vi "Main.vi"(11 "Module Admin":refnum<class "Delacor_lib_QMH_Module Admin.lvclass">) -> ()   [LabVIEW 2020, in "Pruebas.lvlib"]
doc: "This template is based off of the Queued Message Handler design pattern and the Queued Message Handler project template that ships with LabVIEW.\n\nThe main difference is that the queue is private to this module and communication between modules is performed via Broadcast and Request events.\n\nRequest events are wrapped in public API methods and are handled in the Event Handling Loop (EHL) of this VI. Any module can register for Broadcast events sent by this module. The EHL generates messages based on user interface actions.\n\nThe Message Handling Loop (MHL) processes messages generated by the EHL, or by other messages. The messages are string values, so new messages can be added easily to the Message Cases case structure in the MHL. Each message cluster can also provide an optional value for Message Data, which is a variant that can be converted to whatever message-specific data is required.\n_____\nBased on Delacor QMH Project Template 5.0.0.82."
uses:
  Pruebas.lvlib
  <vilib>/Delacor/Delacor QMH/Libraries/Module Admin_class/Delacor_lib_QMH_Module Admin.lvclass
  Module Data--cluster.ctl
  <vilib>/Delacor/Delacor QMH/Libraries/Message Queue_class/Delacor_lib_QMH_Message Queue.lvclass/Delacor_lib_QMH_Message Queue.ctl
  Stop Argument--cluster.ctl
  <vilib>/Delacor/Delacor QMH/Libraries/Module Admin_class/Delacor_lib_QMH_Module Admin.lvclass/Delacor_lib_QMH_Module Admin.ctl
  Mostrar en Subpanel Argument--cluster.ctl
  <vilib>/Utility/miscctls.llb/LVPointTypeDef.ctl
  <vilib>/Delacor/Delacor QMH/Libraries/Message Queue_class/Delacor_lib_QMH_Enqueue Message (Single).vi
  <vilib>/Delacor/Delacor QMH/Libraries/Module Admin_class/Delacor_lib_QMH_Get External Launch.vi
  <vilib>/Utility/error.llb/Error Cluster From Error Code.vi
  <vilib>/ErrorRing/Error Ring.xnode
  <vilib>/Delacor/Delacor QMH/Libraries/Message Queue_class/Delacor_lib_QMH_Message Queue.lvclass
panel:
  out "Señales Debug Ref":refnum<vi>[](array[refnum])
  out "Señales de Prueba Ref":refnum<vi>[](array[refnum])
  in  "Modulación Corrientes":dbl min=0.0 max=50.0 step=5.0 format="%#_g %%"
  in  "Modulación T002":dbl min=0.0 max=90.0 step=5.0 format="%#_g %%"
  in  "Modulación T001":dbl min=0.0 max=90.0 step=5.0 format="%#_g %%"
  in  "DebugMode":bool
  in  "Fases 3 y 4":bool
  in  "Fases 1 y 2":bool
  in  "Cojinetes":bool
  in  "Corriente de Armadura":dbl min=0.0 max=2000.0 step=50.0 format="%#_g A"
  in  "Corriente de Campo":dbl min=0.0 max=3.0 step=0.1 format="%#_g A"
  in  "Tensión Batería":dbl min=0.0 max=340.0 step=10.0 format="%#_g V"
  in  "Tensión Generador":dbl min=0.0 max=340.0 step=10.0 format="%#_g V"
  in  "Habilitar Señales de Prueba":bool
  out "error out":errorcluster
  out "Status":string
  # "Panel de Pruebas"
  # "Depuración [Modulación PWMs]"
  # "Simular Sobretemperatura"
  # "Amperímetros y Voltímetros"
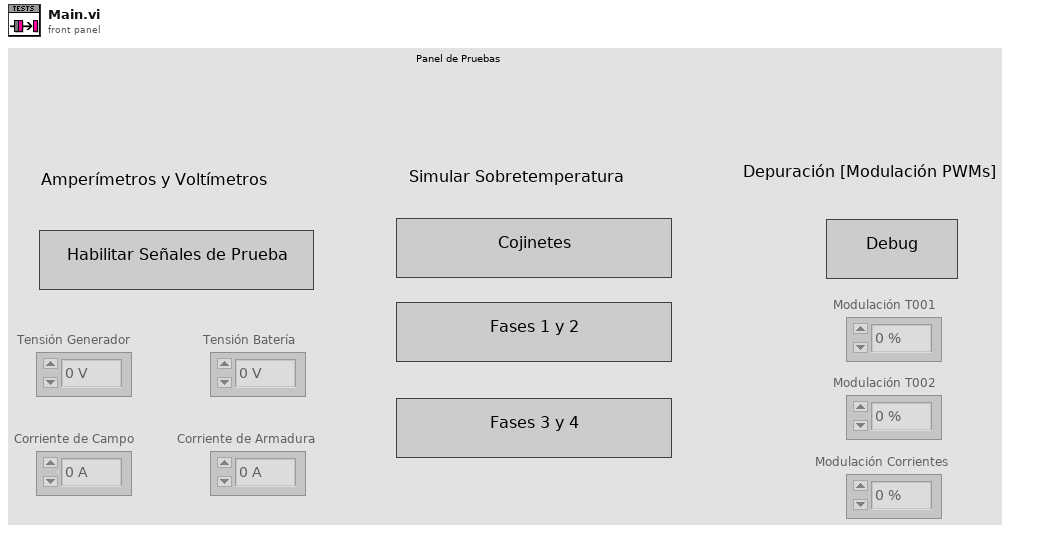
[diagram p1: front panel]
types:
  T1 = typedef "Pruebas.lvlib/Request Events--cluster.ctl" = cluster{"Stop Module":refnum<user-event>, "Show Panel":refnum<user-event>, "Hide Panel":refnum<user-event>, "Get Module Execution Status":refnum<user-event>, "Show Diagram":refnum<user-event>, "Mostrar en Subpanel":refnum<user-event>}
  T2 = typedef "Pruebas.lvlib/Module Data--cluster.ctl" = cluster{"Status":string}
  T3 = enum32{"invalid lock state", "Not Locked", "Locked (No Password)", "Password-protected"}
  T4 = typedef "Pruebas.lvlib/Stop Argument--cluster.ctl" = cluster{"Origin":string, "Exit via Stop Module Req?":bool, "Wait for Module to stop?":bool}
  T5 = typedef "Pruebas.lvlib/Mostrar en Subpanel Argument--cluster.ctl" = cluster{"Subpanel Ref":refnum<vi>}
  T6 = typedef "LVPointTypeDef.ctl" = cluster{"Horizontal":i16, "Vertical":i16}
  T7 = enum32{"Invalid", "Standard", "Closed", "Hidden", "Minimized", "Maximized"}
  T8 = enum8{"Enabled", "Disabled", "Disabled and Grayed Out"}
  T9 = cluster{"Cojinetes":bool, "Fases 1 y 2":bool, "Fases 3 y 4":bool}
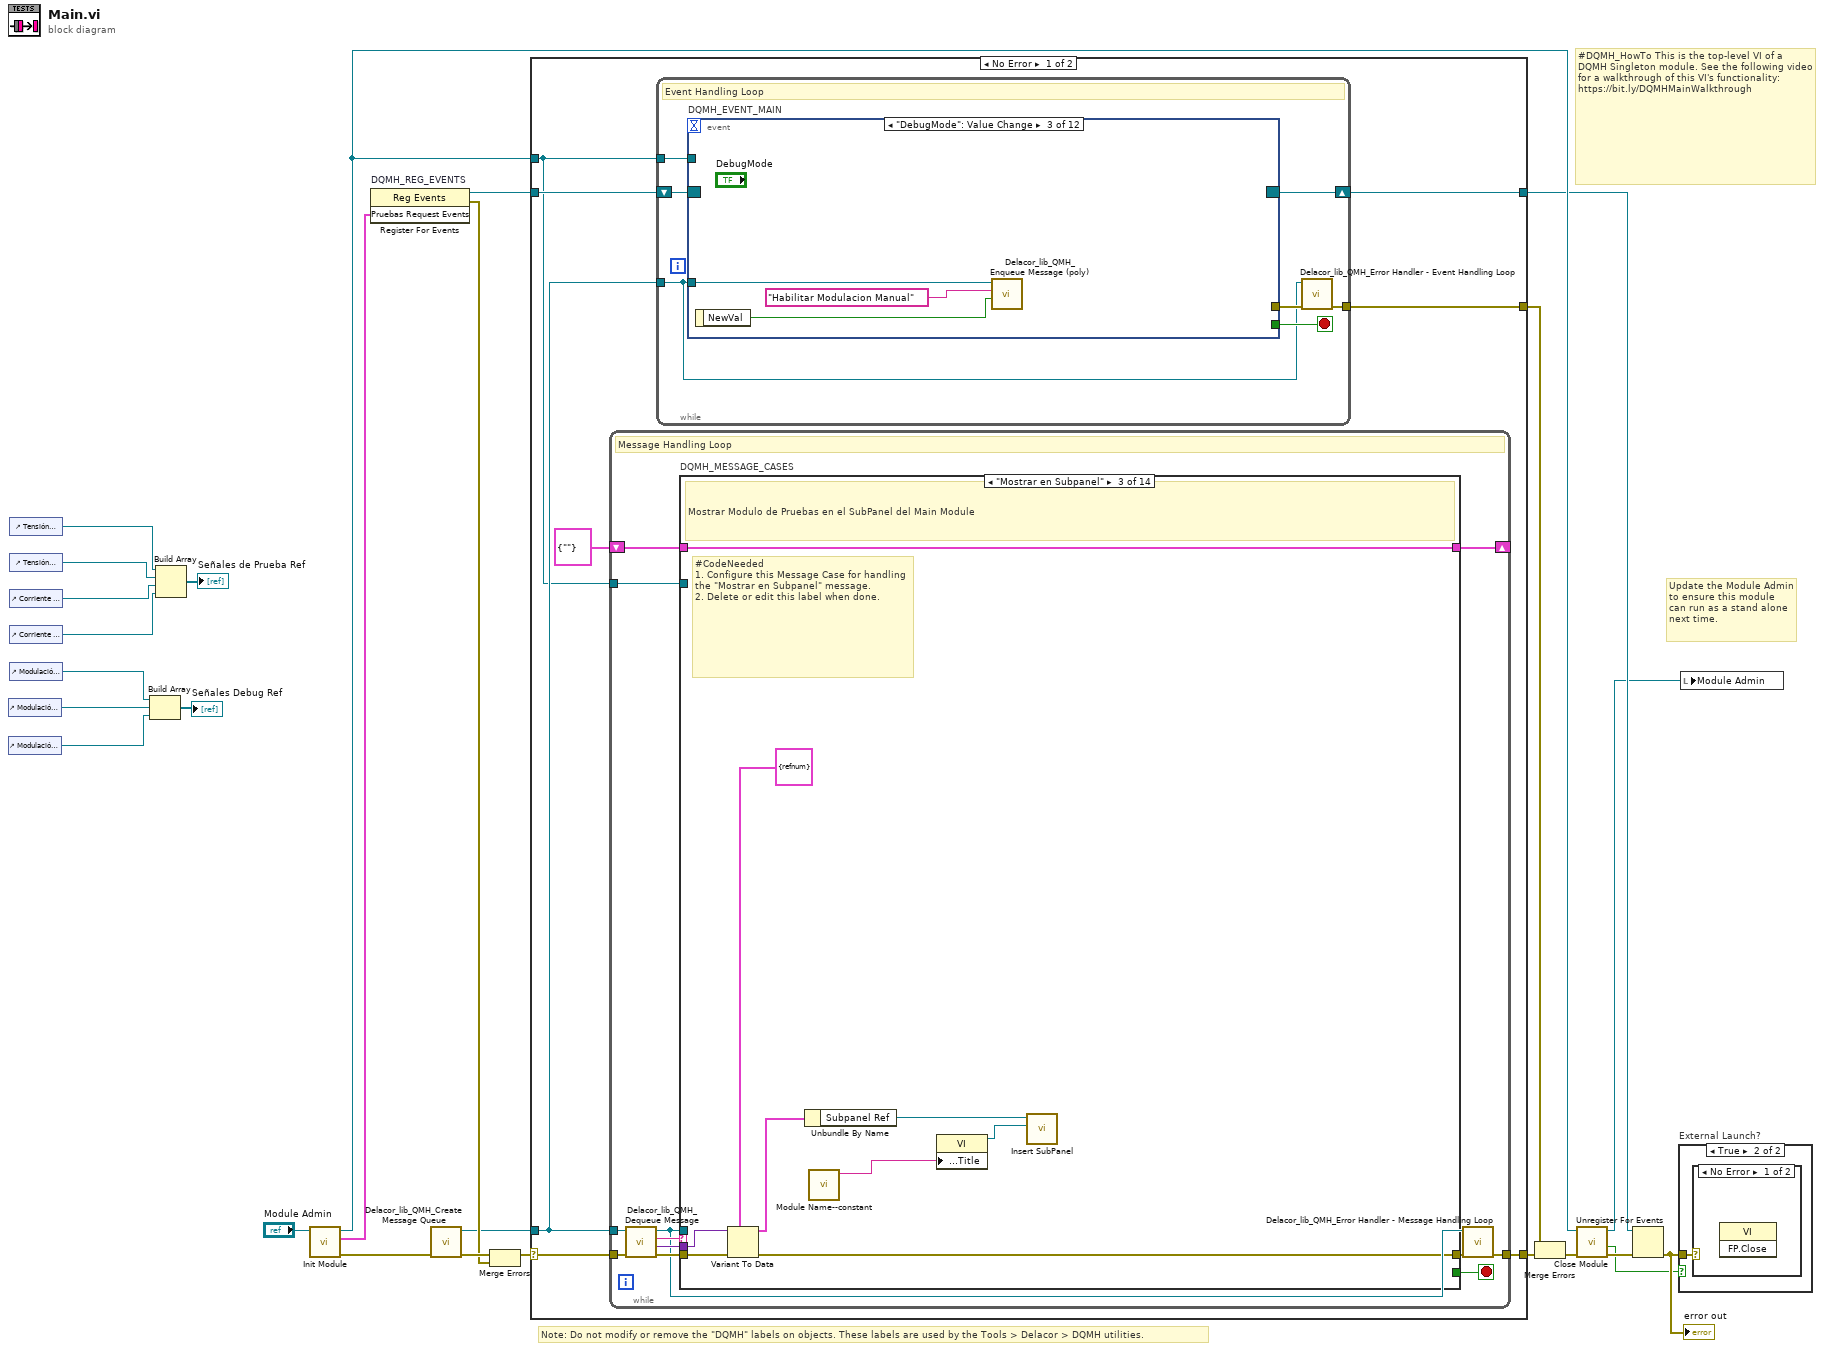
[diagram p0: block diagram]
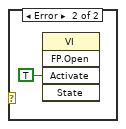
[diagram p3: hidden frame]
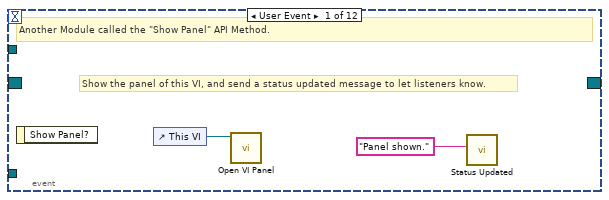
[diagram p4: hidden frame]
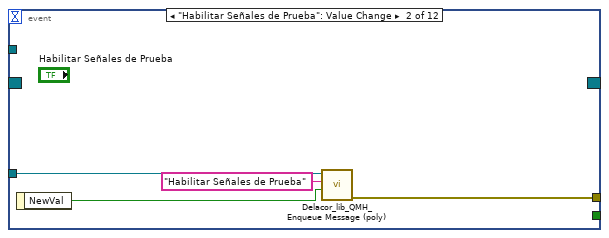
[diagram p5: hidden frame]
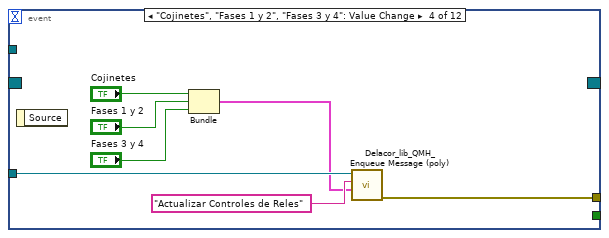
[diagram p6: hidden frame]
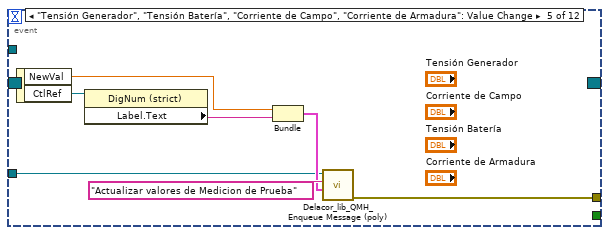
[diagram p7: hidden frame]
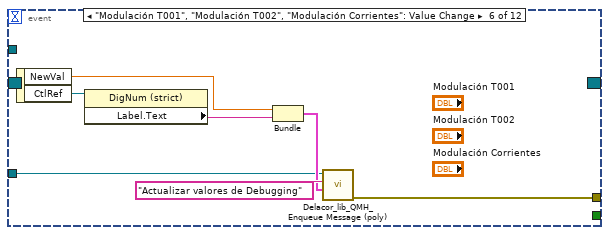
[diagram p8: hidden frame]
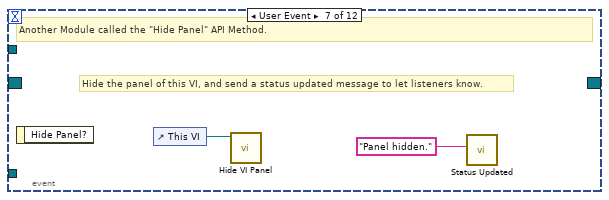
[diagram p9: hidden frame]
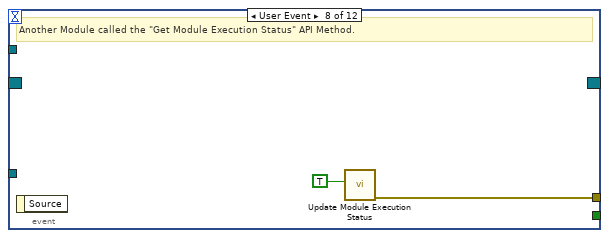
[diagram p10: hidden frame]
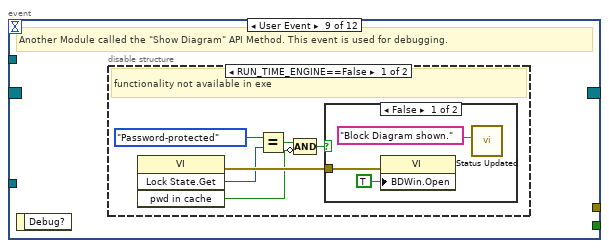
[diagram p11: hidden frame]
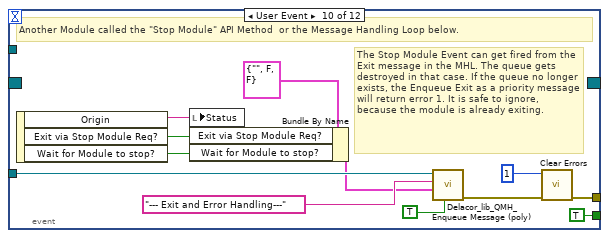
[diagram p14: hidden frame]
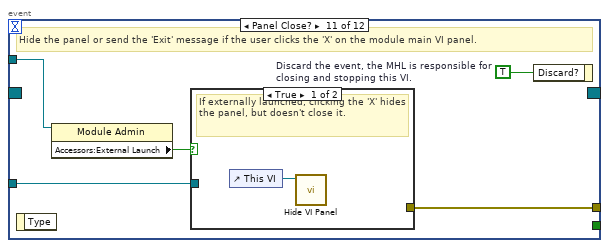
[diagram p15: hidden frame]
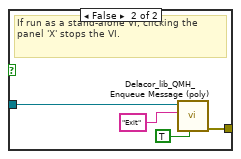
[diagram p16: hidden frame]
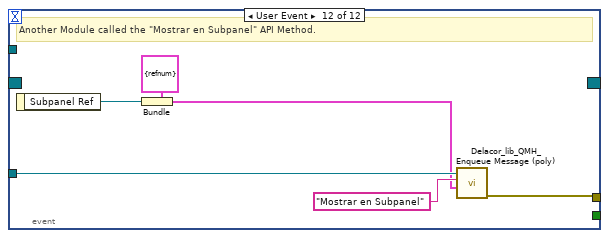
[diagram p17: hidden frame]
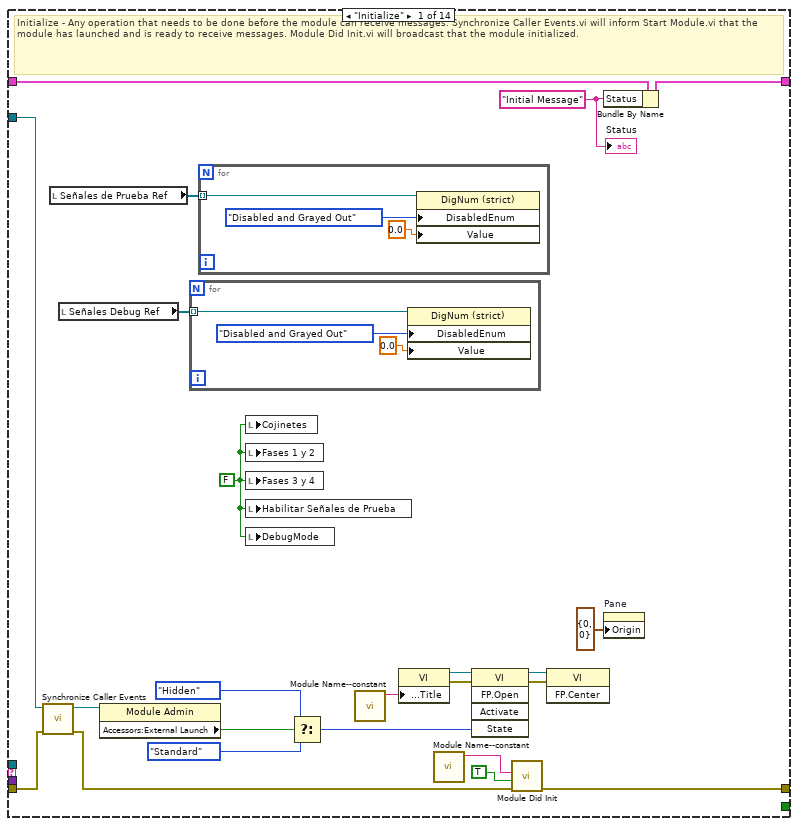
[diagram p18: hidden frame]
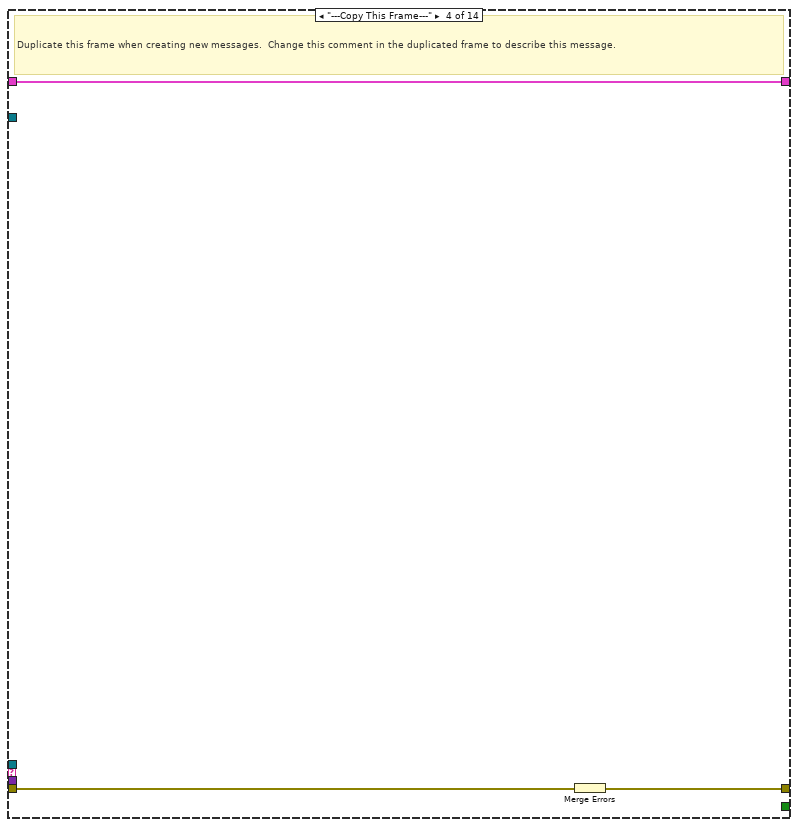
[diagram p20: hidden frame]
diagram:
  # "#DQMH_HowTo This is the top-level VI of a DQMH Singleton module. See the following video for a walkthrough of this VI's functionality: https://bit.ly/DQMHMainWalkthrough"
  # "Note: Do not modify or remove the \"DQMH\" labels on objects. These labels are used by the Tools > Delacor > DQMH utilities."
  # "Update the Module Admin to ensure this module can run as a stand alone next time."
  n1 = control-ref of="Modulación Corrientes"() -> (w3:refnum<vi>)
  n2 = control-ref of="Modulación T002"() -> (w2:refnum<vi>)
  n3 = control-ref of="Tensión Generador"() -> (w9:refnum<vi>)
  n4 = control-ref of="Tensión Batería"() -> (w8:refnum<vi>)
  n5 = control-ref of="Corriente de Campo"() -> (w7:refnum<vi>)
  n6 = control-ref of="Corriente de Armadura"() -> (w6:refnum<vi>)
  n7 = control-ref of="Modulación T001"() -> (w4:refnum<vi>)
  n8 = Build Array(w4, w3, w2) -> (→"Señales Debug Ref":refnum<vi>[])
  n9 = Build Array(w9, w8, w7, w6) -> (→"Señales de Prueba Ref":refnum<vi>[])
  n10 = call "Init Module.vi"("Singleton Module Admin in"="Module Admin") -> ("error out"=w25:errorcluster, "Pruebas Request Events"=w14:T1, "Singleton Module Admin out"=w17:refnum<class "Delacor_lib_QMH_Module Admin.lvclass">)  [unwired: 8 in]
  n11 = register-events "DQMH_REG_EVENTS"(w14) -> (reference out=w15:refnum<event-registration>, error out=w18:errorcluster)  [unwired: 2 in]
  n12 = call <vilib>:"Delacor_lib_QMH_Create Message Queue.vi"("error in"=w25) -> ("error out"=w20:errorcluster, "Message Queue"=w13:refnum<class "Delacor_lib_QMH_Message Queue.lvclass">)  [unwired: 9 in]
  n13 = Merge Errors(w20, w18) -> (w19:errorcluster)
  n14 = case shown="No Error" w19 {
    selector: w19 -> [w32 w309]
    tunnel: [w34 w308] -> w26
    tunnel: [w31 w314] -> w16
    tunnel: w15 -> [w29 w314]
    tunnel: w13 -> [w28 w307]
    tunnel: [w33 _] -> w23
    tunnel: w17 -> [w27 w310]
    frame No Error {
      n15 = while {
        tunnel: w28 -> [w115]
        shift-right: [w119] -> _
        shift-left: T2 {"Status"=""} ("Data Cluster") -> [w120]
        tunnel: w32 -> [w123]
        tunnel: [w121] -> w34
        tunnel: w27 -> [w113]
        stop <- w118 stop-if-true
        # "Message Handling Loop"
        n16 = call-dynamic "Delacor_lib_QMH_Dequeue Message.vi"("error in"=w123, "Message Queue in"=w115) -> ("error out"=w122:errorcluster, "Message Data"=w116:variant, "Message"=w117:string, "Message Queue out"=w114:refnum<class "Delacor_lib_QMH_Message Queue.lvclass">)  [unwired: 6 in]
        n17 = case "DQMH_MESSAGE_CASES" shown="\"Mostrar en Subpanel\"" w117 {
          selector: w117 -> [_ _ _ _ _ _ _ _ _ _ _ _ _ w294]
          tunnel: w114 -> [_ _ _ _ _ _ _ _ _ w247 _ w264 w286 _]
          tunnel: w122 -> [w145 w155 w164 w167 w172 w189 w201 w216 w232 _ w253 w271 w292 w296]
          tunnel: [w143 w155 w162 w166 w175 w192 w204 w219 w235 w246 w252 w267 w289 w297] -> w124
          tunnel: w120 -> [w134 w154 w163 w165 w174 w191 w203 w218 w234 w248 w250 w266 w285 w295]
          tunnel: [w133 w154 w163 w165 w174 w191 w203 w218 w234 w248 w250 w266 w285 w295] -> w119
          tunnel: [_ _ _ _ _ _ _ _ _ _ _ _ w284 _] -> w118
          tunnel: w116 -> [_ _ w161 _ w173 w190 w202 w217 w233 _ _ w265 w283 _]
          tunnel: w113 -> [w135 _ _ _ _ _ _ _ _ _ _ w263 w278 _]
          frame "Initialize" {
            w125 = FALSE ("DebugMode")
            w128 = "Initial Message" ("Initial Message")
            # "Initialize - Any operation that needs to be done before the module can receive messages. Synchronize Caller Events.vi will inform Start Module.vi that the module has launched and is ready to receive messages. Module Did Init.vi will broadcast that the module initialized."
            n18 = call "Synchronize Caller Events.vi"("error in (no error)"=w145, "Singleton Module Admin in"=w135) -> ("error out"=w144:errorcluster, "Singleton Module Admin out"=w130:refnum<class "Delacor_lib_QMH_Module Admin.lvclass">)  [unwired: 8 in]
            n19 = local read "Señales de Prueba Ref"() -> (w127:refnum<vi>[])
            n20 = local read "Señales Debug Ref"() -> (w126:refnum<vi>[])
            n21 = property class="Module Admin"(reference=w130) -> ("Accessors:External Launch"=w139:bool)  [unwired: 1 in, 2 out]
            n22 = for {
              tunnel: w126 -> [w150] mode=indexing
              n23 = property class="DigNum (strict)"(reference=w150, "DisabledEnum"=T8."Disabled and Grayed Out" ("Disabled"), "Value"=0.0) -> ()  [unwired: 1 in, 2 out]
            }
            n24 = for {
              tunnel: w127 -> [w153] mode=indexing
              n25 = property class="DigNum (strict)"(reference=w153, "DisabledEnum"=T8."Disabled and Grayed Out" ("Disabled"), "Value"=0.0) -> ()  [unwired: 1 in, 2 out]
            }
            n26 = local write "Cojinetes"(w125) -> ()
            n27 = local write "Fases 1 y 2"(w125) -> ()
            n28 = local write "Fases 3 y 4"(w125) -> ()
            n29 = local write "Habilitar Señales de Prueba"(w125) -> ()
            n30 = local write "DebugMode"(w125) -> ()
            n31 = Select(t=T7."Hidden" ("State"), s=w139, f=T7."Standard" ("State")) -> (s? t:f=w136:T7)
            n32 = call "Module Name--constant.vi"() -> ("Module Name"=w142:string)  [unwired: 11 in]
            n33 = property class="VI"("Front Panel.Title"=w142) -> (reference out=w141:refnum<vi>, error out=w147:errorcluster)  [unwired: 2 in]
            n34 = call "Module Name--constant.vi"() -> ("Module Name"=w131:string)  [unwired: 11 in]
            n35 = invoke class="VI" method="FP.Open"(reference=w141, error in=w147, "State"=w136) -> (reference out=w140:refnum<vi>, error out=w146:errorcluster)  [unwired: 2 in, 3 out]
            n36 = call "Module Did Init.vi"("error in (no error)"=w144, "Initialized?"=TRUE, "Origin"=w131) -> ("error out"=w143:errorcluster)  [unwired: 8 in]
            n37 = invoke class="VI" method="FP.Center"(reference=w140, error in=w146) -> ()  [unwired: 1 in, 3 out]
            n38 = Bundle By Name(cluster=w134, "Status"=w128) -> (w133:T2)
            n39 = property on="Pane" class="Pane"("Origin"=T6 {"Horizontal"=0, "Vertical"=0}) -> ()  [unwired: 2 in, 2 out]
            "Status" <- w128
          }
          frame "--- Module Specific ---" {
            # "Separator -- The following cases handle messages specific to this Module."
          }
          frame "Mostrar en Subpanel" {
            # "#CodeNeeded\n1. Configure this Message Case for handling the \"Mostrar en Subpanel\" message.\n2. Delete or edit this label when done."
            # "Mostrar Modulo de Pruebas en el SubPanel del Main Module"
            n40 = Variant To Data(error in=w164, type=T5 {"Subpanel Ref"=refnum} ("Mostrar en Subpanel Argument"), Variant=w161) -> (data=w159:T5, error out=w162:errorcluster)
            n41 = Unbundle By Name(w159) -> ("Subpanel Ref"=w158:refnum<vi>)
            n42 = call "Module Name--constant.vi"() -> ("Module Name"=w157:string)  [unwired: 11 in]
            n43 = property class="VI"("Front Panel.Title"=w157) -> (reference out=w156:refnum<vi>)  [unwired: 2 in, 1 out]
            n44 = call "Insert SubPanel.vi"("VI Ref"=w156, "Subpanel Ref"=w158) -> ()  [unwired: 9 in, 1 out]
          }
          frame "---Copy This Frame---" {
            # "Duplicate this frame when creating new messages.  Change this comment in the duplicated frame to describe this message."
            n45 = Merge Errors(w167) -> (w166:errorcluster)
          }
          frame "Habilitar Señales de Prueba" {
            # "Duplicate this frame when creating new messages.  Change this comment in the duplicated frame to describe this message."
            n46 = local read "Señales de Prueba Ref"() -> (w169:refnum<vi>[])
            n47 = Variant To Data(error in=w172, type=FALSE ("Habilitar Señales de Prueba 2"), Variant=w173) -> (data=w168:bool, error out=w171:errorcluster)
            n48 = case shown="True" w168 {
              tunnel: w169 -> [w177 w180]
              frame False {
                w176 = 0.0 ("Tensión Generador")
                n49 = for {
                  tunnel: w177 -> [w179] mode=indexing
                  n50 = property class="DigNum (strict)"(reference=w179, "DisabledEnum"=T8."Disabled and Grayed Out" ("Disabled")) -> ()  [unwired: 1 in, 2 out]
                }
                n51 = local write "Tensión Generador"(w176) -> ()
                n52 = local write "Tensión Batería"(w176) -> ()
                n53 = local write "Corriente de Campo"(w176) -> ()
                n54 = local write "Corriente de Armadura"(w176) -> ()
              }
              frame True {
                n55 = for {
                  tunnel: w180 -> [w182] mode=indexing
                  n56 = property class="DigNum (strict)"(reference=w182, "DisabledEnum"=T8."Enabled" ("Disabled")) -> ()  [unwired: 1 in, 2 out]
                }
              }
            }
            n57 = Merge Errors(w171) -> (w175:errorcluster)
          }
          frame "Actualizar valores de Medicion de Prueba" {
            # "Duplicate this frame when creating new messages.  Change this comment in the duplicated frame to describe this message."
            n58 = Variant To Data(error in=w189, type=cluster{"NewVal":dbl, "Label.Text":string} {"NewVal"=0.0, "Label.Text"=""} ("output cluster"), Variant=w190) -> (data=w187:cluster{"NewVal":dbl, "Label.Text":string}, error out=w184:errorcluster)
            n59 = Unbundle(w187) -> ("NewVal"=w186:dbl, "Label.Text"=w185:string)
            n60 = call "Valor de Medicion de Prueba Enviado.vi"("error in (no error)"=w184, "Nombre del Valor"=w185, "Valor"=w186) -> ("error out"=w183:errorcluster)  [unwired: 8 in]
            n61 = Merge Errors(w183) -> (w192:errorcluster)
          }
          frame "Actualizar valores de Debugging" {
            # "Duplicate this frame when creating new messages.  Change this comment in the duplicated frame to describe this message."
            n62 = Variant To Data(error in=w201, type=cluster{"NewVal":dbl, "Label.Text":string} {"NewVal"=0.0, "Label.Text"=""} ("output cluster"), Variant=w202) -> (data=w199:cluster{"NewVal":dbl, "Label.Text":string}, error out=w197:errorcluster)
            n63 = Unbundle(w199) -> ("NewVal"=w195:dbl, "Label.Text"=w196:string)
            n64 = Divide(x=w195, y=100.0) -> (x/y=w194:dbl)
            n65 = case shown="\"Modulación T001\"" w196 {
              tunnel: w194 -> [w206 w208 w210]
              frame "Modulación T002", Default {
                n66 = shared-variable-write(refnum<k21> "ni.var.psp://EmuGenV2/VariablesEmuGenV2/Mod T002 Debug" ("shared variable refnum in"), w206) -> ()  [unwired: 1 in, 2 out]
              }
              frame "Modulación Corrientes" {
                n67 = shared-variable-write(refnum<k21> "ni.var.psp://EmuGenV2/VariablesEmuGenV2/Mod Corriente Debug" ("shared variable refnum in"), w208) -> ()  [unwired: 1 in, 2 out]
              }
              frame "Modulación T001" {
                n68 = shared-variable-write(refnum<k21> "ni.var.psp://EmuGenV2/VariablesEmuGenV2/Mod T001 Debug" ("shared variable refnum in"), w210) -> ()  [unwired: 1 in, 2 out]
              }
            }
            n69 = call "Valor de Modulacion Debugging Enviado.vi"("error in (no error)"=w197, "Nombre"=w196, "Valor"=w195) -> ("error out"=w198:errorcluster)  [unwired: 8 in]
            n70 = Merge Errors(w198) -> (w204:errorcluster)
          }
          frame "Habilitar Modulacion Manual" {
            # "Duplicate this frame when creating new messages.  Change this comment in the duplicated frame to describe this message."
            n71 = local read "Señales Debug Ref"() -> (w213:refnum<vi>[])
            n72 = Variant To Data(error in=w216, type=FALSE ("Habilitar Señales de Prueba 2"), Variant=w217) -> (data=w212:bool, error out=w215:errorcluster)
            n73 = case shown="True" w212 {
              tunnel: w213 -> [w220 w223]
              frame False {
                n74 = for {
                  tunnel: w220 -> [w222] mode=indexing
                  n75 = property class="DigNum (strict)"(reference=w222, "DisabledEnum"=T8."Disabled and Grayed Out" ("Disabled")) -> ()  [unwired: 1 in, 2 out]
                }
              }
              frame True {
                n76 = for {
                  tunnel: w223 -> [w225] mode=indexing
                  n77 = property class="DigNum (strict)"(reference=w225, "DisabledEnum"=T8."Enabled" ("Disabled")) -> ()  [unwired: 1 in, 2 out]
                }
              }
            }
            n78 = shared-variable-write(refnum<k21> "ni.var.psp://EmuGenV2/VariablesEmuGenV2/Habilitar Debug" ("shared variable refnum in"), w212) -> ()  [unwired: 1 in, 2 out]
            n79 = Merge Errors(w215) -> (w219:errorcluster)
          }
          frame "Actualizar Controles de Reles" {
            # "Duplicate this frame when creating new messages.  Change this comment in the duplicated frame to describe this message."
            n80 = Variant To Data(error in=w232, type=T9 {"Cojinetes"=FALSE, "Fases 1 y 2"=FALSE, "Fases 3 y 4"=FALSE} ("output cluster"), Variant=w233) -> (data=w229:T9, error out=w231:errorcluster)
            n81 = Unbundle By Name(w229) -> ("Fases 3 y 4"=w228:bool, "Cojinetes"=w227:bool, "Fases 1 y 2"=w226:bool)
            n82 = call "Controles de relés de prueba actualizados.vi"("Fases 3 y 4"=w228, "Fases 1 y 2"=w226, "Cojinete"=w227) -> ()  [unwired: 8 in, 1 out]
            n83 = Merge Errors(w231) -> (w235:errorcluster)
          }
          frame "--- Exit and Error Handling---" {
            # "Separator - The following cases handle errors and exit messages."
            n84 = call-poly <vilib>:"Delacor_lib_QMH_Enqueue Message (poly).vi"("Message Data"=T4 {"Origin"="", "Exit via Stop Module Req?"=FALSE, "Wait for Module to stop?"=FALSE} ("Stop Argument"), "Message"="Exit", "Message Queue in"=w247) -> ("error out"=w246:errorcluster)  [unwired: 7 in, 1 out]
            n85 = shared-variable-write(refnum<k21> "ni.var.psp://EmuGenV2/VariablesEmuGenV2/Habilitar Debug" ("shared variable refnum in"), FALSE ("Habilitar Debug")) -> ()  [unwired: 1 in, 2 out]
            n86 = shared-variable-write(refnum<k21> "ni.var.psp://EmuGenV2/VariablesEmuGenV2/Mod T001 Debug" ("shared variable refnum in"), 0.0 ("Mod T001 Debug")) -> ()  [unwired: 1 in, 2 out]
            n87 = shared-variable-write(refnum<k21> "ni.var.psp://EmuGenV2/VariablesEmuGenV2/Mod T002 Debug" ("shared variable refnum in"), 0.0 ("Mod T002 Debug")) -> ()  [unwired: 1 in, 2 out]
            n88 = shared-variable-write(refnum<k21> "ni.var.psp://EmuGenV2/VariablesEmuGenV2/Mod Corriente Debug" ("shared variable refnum in"), 0.0 ("Mod Corriente Debug")) -> ()  [unwired: 1 in, 2 out]
          }
          frame "Simulate MHL Error" {
            # "#DQMH_HowTo The 'Simulate MHL Error' button  illustrates how the MHL handles errors. This event is instructional in nature and can be removed."
            # "Simulate an error occurring at the MHL"
            n89 = call "Module Name--constant.vi"() -> ("Module Name"=w249:string)  [unwired: 11 in]
            n90 = xnode "Error Ring"("parameter 0"=w249) -> ("error out"=w251:errorcluster)
            n91 = Merge Errors(w253, w251) -> (w252:errorcluster)
          }
          frame "Error" {
            # "#CodeRecommended - If you ever change the name of this \"Error\" message, you'll need to update the name in the Check Loop Error.vi as well."
            # "#CodeRecommended - If the module is running in standalone mode (External Launch = FALSE), this code will pop up an error dialog and call the 'Exit' message if an error occurs. Add more fine-grained error handling here."
            # "Error - Check the error message data and respond accordingly. This message is sent by the \"Error Handler\" VIs at the end of each loop in this application."
            n92 = property class="Module Admin"(reference=w263) -> ("Accessors:External Launch"=w262:bool)  [unwired: 1 in, 2 out]
            n93 = Variant To Data(error in=w271, type=errorcluster {"status"=FALSE, "code"=0, "source"=""} ("error constant"), Variant=w265) -> (data=w272:errorcluster, error out=w269:errorcluster)
            n94 = call "Module Name--constant.vi"() -> ("Module Name"=w261:string)  [unwired: 11 in]
            n95 = call "Error Reported.vi"("Additional Information"=w261, "Error"=w272) -> ()  [unwired: 9 in, 1 out]
            n96 = case shown="False" w262 {
              tunnel: [w277 _] -> w268
              tunnel: w264 -> [w275 _]
              tunnel: w272 -> [w276 _]
              frame False {
                # "If the module is running standalone, then pop up an error dialog and call the \"Exit\" message."
                n97 = call <vilib>:"Simple Error Handler.vi"("error in (no error)"=w276) -> ()  [unwired: 4 in, 5 out]
                n98 = call-poly <vilib>:"Delacor_lib_QMH_Enqueue Message (poly).vi"("Priority Message? (F)"=TRUE, "Message"="Exit", "Message Queue in"=w275) -> ("error out"=w277:errorcluster)  [unwired: 7 in, 1 out]
              }
              frame True {
                # "If the module was launched externally, calling the Error Reported broadcast VI is the only action performed by the \"Error\" message. The module's caller can then process the error appropriately."
              }
            }
            n99 = Merge Errors(w269, w268) -> (w267:errorcluster)
            n100 = local write "error out"(w267) -> ()
          }
          frame "Exit" {
            w282 = 91  # 91: not all Exit messages will have an argument
            w284 = TRUE  # Stop the VI
            # "Release the message queue reference"
            # "#CodeNeeded - Add any required cleanup code here"
            # "Exit - Exit the application."
            n101 = Variant To Data(error in=w292, type=T4 {"Origin"="", "Exit via Stop Module Req?"=FALSE, "Wait for Module to stop?"=FALSE} ("Stop Argument"), Variant=w283) -> (data=w280:T4, error out=w288:errorcluster)
            n102 = call <vilib>:"Clear Errors.vi"("error in (no error)"=w288, "specific error code to clear (0: all)"=w282) -> ("error out"=w291:errorcluster)  [unwired: 4 in, 1 out]
            n103 = control-ref of="This VI"() -> (w279:refnum<vi>)
            n104 = call-dynamic "Delacor_lib_QMH_Release Message Queue.vi"("error in"=w291, "Message Queue"=w286) -> ("error out"=w290:errorcluster)  [unwired: 9 in]
            n105 = call "Handle Exit.vi"("Stop Argument"=w280, "Admin in"=w278, "VI reference"=w279) -> ("error out"=w287:errorcluster)  [unwired: 7 in, 1 out]
            n106 = Merge Errors(w290, w287) -> (w289:errorcluster)
          }
          frame Default {
            # "'Default' case only runs if there is a message that isn't defined in any of the other cases.  Output a programming error."
            n107 = call "Module Name--constant.vi"() -> ("Module Name"=w293:string)  [unwired: 11 in]
            n108 = xnode "Error Ring"("parameter 0"=w294, "parameter 1"=w293) -> ("error out"=w298:errorcluster)
            n109 = Merge Errors(w296, w298) -> (w297:errorcluster)
          }
        }
        n110 = call-dynamic "Delacor_lib_QMH_Error Handler - Message Handling Loop.vi"("error in"=w124, "Message Queue in"=w114) -> ("dup error in"=w121:errorcluster)  [unwired: 8 in, 1 out]
      }
      n111 = while {
        tunnel: w28 -> [w35]
        shift-right: [w38] -> w31
        shift-left: w29 -> [w39]
        tunnel: [w40] -> w33
        tunnel: w27 -> [w36]
        stop <- w37 stop-if-true
        # "Event Handling Loop"
        n112 = event "DQMH_EVENT_MAIN" shown="[2] \"DebugMode\": Value Change" {
          selector: w39 -> [_ _ _ _ _ _ _ _ _ _ _ _]
          dyn-events: [_ _ _ _ _ _ _ _ _ _ _ _] -> w38
          timeout: _ -> [_ _ _ _ _ _ _ _ _ _ _ _]
          tunnel: [_ _ _ _ _ _ _ _ _ TRUE ("Discard?") _ _] -> w37
          tunnel: w35 -> [_ w47 w49 w57 w59 w66 _ _ _ w92 w99 w112]
          tunnel: [_ w46 _ w51 w58 w65 _ w75 _ w95 w101 w107] -> w41
          tunnel: w36 -> [_ _ _ _ _ _ _ _ _ _ w98 _]
          event User Event {
            # "Show the panel of this VI, and send a status updated message to let listeners know."
            # "Another Module called the \"Show Panel\" API Method."
            n113 = event-data() -> ()  [unwired: 1 in, 1 out]
            n114 = control-ref of="This VI"() -> (w43:refnum<vi>)
            n115 = call "Open VI Panel.vi"("VI"=w43) -> ()  [unwired: 10 in, 1 out]
            n116 = call "Status Updated.vi"("Status"="Panel shown." ("format string")) -> ()  [unwired: 10 in, 1 out]
          }
          event "Habilitar Señales de Prueba": Value Change {
            n117 = event-data() -> ("NewVal"=w44:bool)  [unwired: 1 in]
            n118 = call-poly <vilib>:"Delacor_lib_QMH_Enqueue Message (poly).vi"("Message Data"=w44, "Message"="Habilitar Señales de Prueba", "Message Queue in"=w47) -> ("error out"=w46:errorcluster)  [unwired: 7 in, 1 out]
          }
          event "DebugMode": Value Change {
            n119 = event-data() -> ("NewVal"=w48:bool)  [unwired: 1 in]
            n120 = call-poly <vilib>:"Delacor_lib_QMH_Enqueue Message (poly).vi"("Message Data"=w48, "Message"="Habilitar Modulacion Manual", "Message Queue in"=w49) -> ()  [unwired: 7 in, 2 out]
          }
          event "Cojinetes", "Fases 1 y 2", "Fases 3 y 4": Value Change {
            n121 = event-data() -> ()  [unwired: 1 in, 1 out]
            n122 = Bundle("Cojinetes"="Cojinetes", "Fases 1 y 2"="Fases 1 y 2", "Fases 3 y 4"="Fases 3 y 4") -> (w52:T9)  [unwired: 1 in]
            n123 = call-poly <vilib>:"Delacor_lib_QMH_Enqueue Message (poly).vi"("Message Data"=w52, "Message"="Actualizar Controles de Reles", "Message Queue in"=w57) -> ("error out"=w51:errorcluster)  [unwired: 7 in, 1 out]
          }
          event "Tensión Generador", "Tensión Batería", "Corriente de Campo", "Corriente de Armadura": Value Change {
            n124 = event-data() -> ("NewVal"=w62:dbl, "CtlRef"=w64:refnum<vi>)  [unwired: 1 in]
            n125 = property class="DigNum (strict)"(reference=w64) -> ("Label.Text"=w61:string)  [unwired: 1 in, 2 out]
            n126 = Bundle("NewVal"=w62, "Label.Text"=w61) -> (w60:cluster{"NewVal":dbl, "Label.Text":string})  [unwired: 1 in]
            n127 = call-poly <vilib>:"Delacor_lib_QMH_Enqueue Message (poly).vi"("Message Data"=w60, "Message"="Actualizar valores de Medicion de Prueba", "Message Queue in"=w59) -> ("error out"=w58:errorcluster)  [unwired: 7 in, 1 out]
          }
          event "Modulación T001", "Modulación T002", "Modulación Corrientes": Value Change {
            n128 = event-data() -> ("NewVal"=w69:dbl, "CtlRef"=w71:refnum<vi>)  [unwired: 1 in]
            n129 = property class="DigNum (strict)"(reference=w71) -> ("Label.Text"=w68:string)  [unwired: 1 in, 2 out]
            n130 = Bundle("NewVal"=w69, "Label.Text"=w68) -> (w67:cluster{"NewVal":dbl, "Label.Text":string})  [unwired: 1 in]
            n131 = call-poly <vilib>:"Delacor_lib_QMH_Enqueue Message (poly).vi"("Message Data"=w67, "Message"="Actualizar valores de Debugging", "Message Queue in"=w66) -> ("error out"=w65:errorcluster)  [unwired: 7 in, 1 out]
          }
          event User Event {
            # "Hide the panel of this VI, and send a status updated message to let listeners know."
            # "Another Module called the \"Hide Panel\" API Method."
            n132 = event-data() -> ()  [unwired: 1 in, 1 out]
            n133 = control-ref of="This VI"() -> (w73:refnum<vi>)
            n134 = call "Hide VI Panel.vi"("VI"=w73) -> ()  [unwired: 10 in, 1 out]
            n135 = call "Status Updated.vi"("Status"="Panel hidden." ("format string")) -> ()  [unwired: 10 in, 1 out]
          }
          event User Event {
            # "Another Module called the \"Get Module Execution Status\" API Method."
            n136 = event-data() -> ()  [unwired: 1 in, 1 out]
            n137 = call "Update Module Execution Status.vi"("Running?"=TRUE) -> ("error out"=w75:errorcluster)  [unwired: 10 in]
          }
          event User Event {
            # "Another Module called the \"Show Diagram\" API Method. This event is used for debugging."
            n138 = event-data() -> ()  [unwired: 1 in, 1 out]
            n139 = disable-structure shown="RUN_TIME_ENGINE==False" {
              frame condition #0 (active) {
                # "functionality not available in exe"
                n140 = invoke class="VI" method="Lock State.Get"() -> (error out=w81:errorcluster, "Get Lock State"=w80:T3, "pwd in cache"=w77:bool)  [unwired: 4 in, 1 out]
                n141 = Equal?(x=T3."Password-protected", y=w80) -> (x = y?=w78:bool)
                n142 = Compound Arithmetic op=AND(w78, invert w77) -> (w76:bool)
                n143 = case shown="False" w76 {
                  tunnel: w81 -> [w84 _]
                  frame False {
                    n144 = property class="VI"(error in=w84, "BDWin.Open"=TRUE ("Block Diagram Window:Open")) -> ()  [unwired: 1 in, 2 out]
                    n145 = call "Status Updated.vi"("Status"="Block Diagram shown." ("format string")) -> ()  [unwired: 10 in, 1 out]
                  }
                  frame True {
                    # "Password-protected VI, and the password is not in the cache. Do not show the diagram."
                  }
                }
              }
              frame condition #1 {
              }
            }
          }
          event User Event {
            # "The Stop Module Event can get fired from the Exit message in the MHL. The queue gets destroyed in that case. If the queue no longer exists, the Enqueue Exit as a priority message will return error 1. It is safe to ignore, because the module is already exiting."
            # "Another Module called the \"Stop Module\" API Method  or the Message Handling Loop below."
            n146 = event-data() -> ("Origin"=w91:string, "Exit via Stop Module Req?"=w87:bool, "Wait for Module to stop?"=w86:bool)  [unwired: 1 in]
            n147 = local write "Status"(w91) -> ()
            n148 = Bundle By Name(cluster=T4 {"Origin"="", "Exit via Stop Module Req?"=FALSE, "Wait for Module to stop?"=FALSE} ("Stop Argument"), "Exit via Stop Module Req?"=w87, "Wait for Module to stop?"=w86) -> (w85:T4)
            n149 = call-poly <vilib>:"Delacor_lib_QMH_Enqueue Message (poly).vi"("Priority Message? (F)"=TRUE, "Message Data"=w85, "Message"="--- Exit and Error Handling---", "Message Queue in"=w92) -> ("error out"=w96:errorcluster)  [unwired: 6 in, 1 out]
            n150 = call <vilib>:"Clear Errors.vi"("error in (no error)"=w96, "specific error code to clear (0: all)"=1) -> ("error out"=w95:errorcluster)  [unwired: 4 in, 1 out]
          }
          event Panel Close? {
            w100 = TRUE  # Discard the event, the MHL is responsible for closing and stopping this VI.
            # "Hide the panel or send the 'Exit' message if the user clicks the 'X' on the module main VI panel."
            n151 = event-data() -> ()  [unwired: 1 in, 1 out]
            n152 = property class="Module Admin"(reference=w98) -> ("Accessors:External Launch"=w97:bool)  [unwired: 1 in, 2 out]
            n153 = case shown="True" w97 {
              tunnel: w99 -> [_ w105]
              tunnel: [_ w106] -> w101
              frame True {
                # "If externally launched, clicking the 'X' hides the panel, but doesn't close it."
                n154 = control-ref of="This VI"() -> (w102:refnum<vi>)
                n155 = call "Hide VI Panel.vi"("VI"=w102) -> ()  [unwired: 10 in, 1 out]
              }
              frame False {
                # "If run as a stand-alone VI, clicking the panel 'X' stops the VI."
                n156 = call-poly <vilib>:"Delacor_lib_QMH_Enqueue Message (poly).vi"("Priority Message? (F)"=TRUE, "Message"="Exit", "Message Queue in"=w105) -> ("error out"=w106:errorcluster)  [unwired: 7 in, 1 out]
              }
            }
            n157 = event-data("Discard?"=w100) -> ()  [unwired: 1 in, 1 out]
          }
          event User Event {
            # "Another Module called the \"Mostrar en Subpanel\" API Method."
            n158 = event-data() -> ("Subpanel Ref"=w108:refnum<vi>)  [unwired: 1 in]
            n159 = Bundle(cluster=T5 {"Subpanel Ref"=refnum} ("Mostrar en Subpanel Argument"), "Subpanel Ref"=w108) -> (w109:T5)
            n160 = call-poly <vilib>:"Delacor_lib_QMH_Enqueue Message (poly).vi"("Message Data"=w109, "Message"="Mostrar en Subpanel", "Message Queue in"=w112) -> ("error out"=w107:errorcluster)  [unwired: 7 in, 1 out]
          }
        }
        n161 = call-dynamic "Delacor_lib_QMH_Error Handler - Event Handling Loop.vi"("error in"=w41, "Message Queue in"=w35) -> ("dup error in"=w40:errorcluster)  [unwired: 8 in, 1 out]
      }
    }
    frame Error {
      # "Synchronize Caller Events.vi will inform Start Module.vi that the module has launched and will let the code calling Start Module.vi register for broadcasts and would permit the caller receive the broadcast that an error occurred at launch time."
      n162 = call-dynamic "Delacor_lib_QMH_Release Message Queue.vi"("error in"=w309, "Message Queue"=w307) -> ("error out"=w308:errorcluster)  [unwired: 9 in]
      n163 = call "Synchronize Caller Events.vi"("Singleton Module Admin in"=w310) -> ("error out"=w315:errorcluster)  [unwired: 9 in, 1 out]
      n164 = call "Module Name--constant.vi"() -> ("Module Name"=w313:string)  [unwired: 11 in]
      n165 = Format Into String(format string="An error occurred during initialization. %s is no longer running.", w313) -> (resulting string=w311:string)  [unwired: 2 in, 1 out]
      n166 = Merge Errors(w308, w315) -> (w316:errorcluster)
      n167 = call "Error Reported.vi"("Additional Information"=w311, "Error"=w316) -> ()  [unwired: 9 in, 1 out]
    }
  }
  n168 = Merge Errors(w23, w26) -> (w22:errorcluster)
  n169 = call "Close Module.vi"("error in (no error)"=w22, "Module Admin in"=w17) -> ("error out"=w24:errorcluster, "External Launch"=w10:bool, "Module Admin out"=w11:refnum<class "Delacor_lib_QMH_Module Admin.lvclass">)  [unwired: 7 in]
  n170 = Unregister For Events(event registration refnum=w16, error in=w24) -> (error out=w21:errorcluster)
  "error out" <- w21
  n171 = case "External Launch?" shown="True" w10 {
    tunnel: w21 -> [_ w317]
    frame False {
    }
    frame True {
      n172 = case shown="No Error" w317 {
        frame No Error {
          n173 = invoke class="VI" method="FP.Close"() -> ()  [unwired: 3 in, 3 out]
        }
        frame Error {
          n174 = invoke class="VI" method="FP.Open"("Activate"=TRUE ("Activate?")) -> ()  [unwired: 4 in, 5 out]
        }
      }
    }
  }
  n175 = local write "Module Admin"(w11) -> ()
